vi "XY Graph Set X Scales Grid Colors.vi"(8 "error in (no error)":errorcluster, 10 "Array of Grid Colors":T2[](array[typedef]), 11 "XYGraph in":T1) -> (0 "error out":errorcluster, 3 "XYGraph out":T1)   [LabVIEW 2021, in "XY Graph Add-Ons.lvlib"]
uses:
  XY Graph Add-Ons.lvlib
  XY Graph Refnum.ctl
  <vilib>/Utility/miscctls.llb/LVMajorAndMinorColorsTypeDef.ctl
  XY Graph Property Tag List.ctl
  <vilib>/UserTags/UserTags.lvlib
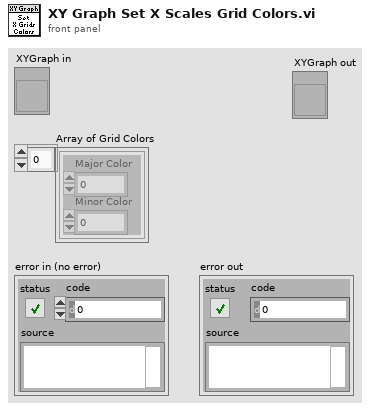
[diagram p1: front panel]
types:
  T1 = typedef "XY Graph Add-Ons.lvlib/XY Graph Refnum.ctl" = refnum<vi>
  T2 = typedef "LVMajorAndMinorColorsTypeDef.ctl" = cluster{"Major Color":u32, "Minor Color":u32}
  T3 = typedef "XY Graph Add-Ons.lvlib/XY Graph Property Tag List.ctl" = enum16{"Max Legend Size", "Preserved Plots", "XScales.GridColors", "YScales.GridColors", "TipStrip String", "TipStrip Visible", "Tool Panels Visibility", "Plots Metadata"}
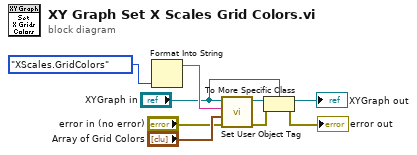
[diagram p0: block diagram]
diagram:
  n1 = Format Into String(XY_Graph_Property_Tag_List."XScales.GridColors" ("XY Graph Property Tag")) -> (resulting string=w9:string)  [unwired: 3 in, 1 out]
  n2 = call <vilib>:"Set User Object Tag.vi"("error in (no error)"="error in (no error)", "Value"="Array of Grid Colors", "Tag Name"=w9, "Generic Refnum"="XYGraph in") -> ("error out"=w2:errorcluster, "dup Generic Refnum"=w5:refnum<vi>)  [unwired: 5 in, 1 out]
  n3 = To More Specific Class(target class="XYGraph in", reference=w5, error in=w2) -> (specific class reference=→"XYGraph out":T1, error out=→"error out":errorcluster)
